vi "P10.vi"() -> ()   [LabVIEW 2019]
panel:
  out "Final Position":dbl
  out "Loop Sum":i32
  in  "stop":bool
  in  "Initial Position":dbl
  in  "error in (no error)":errorcluster
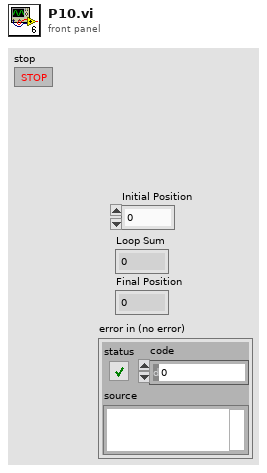
[diagram p1: front panel]
types:
  T1 = enum16{"Initial Position", "Process 1", "Process 2", "Read"}
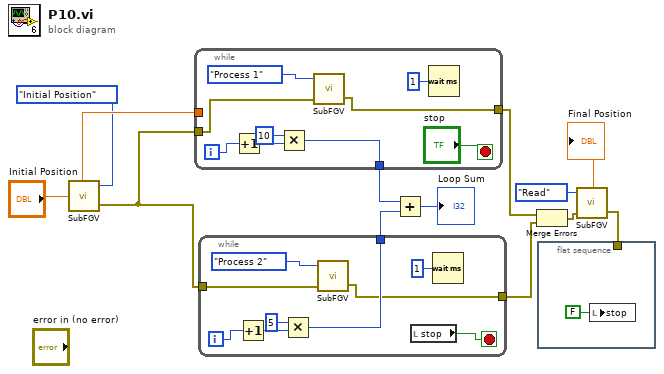
[diagram p0: block diagram]
diagram:
  n1 = call "SubFGV.vi"("Initial Position"="Initial Position", "Enum"=T1."Initial Position") -> ("error out"=w12:errorcluster, "New Position"=w13:dbl)  [unwired: 1 in]
  n2 = while {
    tunnel: [w18] -> w10
    tunnel: w13 -> [_]
    tunnel: w12 -> [w15]
    tunnel: [w14] -> w4
    i -> [w21]
    stop <- "stop" stop-if-true
    n3 = Increment(x=w21) -> (x+1=w20:i32)
    n4 = Multiply(x=10, y=w20) -> (x*y=w18:i32)
    n5 = call "SubFGV.vi"("error in (no error)"=w15, "Enum"=T1."Process 1") -> ("error out"=w14:errorcluster)  [unwired: 1 in, 1 out]
    n6 = Wait (ms)(milliseconds to wait=u32 1) -> ()  [unwired: 1 out]
  }
  n7 = while {
    tunnel: [w27] -> w11
    tunnel: [w25] -> w3
    tunnel: w12 -> [w24]
    i -> [w30]
    stop <- w23 stop-if-true
    n8 = Increment(x=w30) -> (x+1=w29:i32)
    n9 = Multiply(x=5, y=w29) -> (x*y=w27:i32)
    n10 = call "SubFGV.vi"("error in (no error)"=w24, "Enum"=T1."Process 2") -> ("error out"=w25:errorcluster)  [unwired: 1 in, 1 out]
    n11 = local read "stop"() -> (w23:bool)
    n12 = Wait (ms)(milliseconds to wait=u32 1) -> ()  [unwired: 1 out]
  }
  n13 = Add(x=w10, y=w11) -> (x+y=→"Loop Sum":i32)
  n14 = Merge Errors(w4, w3) -> (w5:errorcluster)
  n15 = flat-sequence {
    tunnel: w7 -> [_]
    frame #0 {
      n16 = local write "stop"(FALSE ("stop")) -> ()
    }
  }
  n17 = call "SubFGV.vi"("error in (no error)"=w5, "Enum"=T1."Read") -> ("error out"=w7:errorcluster, "New Position"=→"Final Position":dbl)  [unwired: 1 in]
